vi "Base Card Passthrough(Relay).vi"(4 "Iterations":u32=50 min=1 max=64, 6 "Channels (1-64)":u16=64 min=1 max=64, 9 "Disconnection":enum16{"Open All", "Disconnect All"}(ring)=enum."Disconnect All", 11 "device":refnum<k21>="SET-2010-Mod2") -> (0 "error out":errorcluster, 1 "Disconnect Timing":T1, 2 "Connect Timing":T1)   [LabVIEW 2020, in "slsc-switch-benchmarks.lvlib"]
uses:
  slsc-switch-benchmarks.lvlib
  Timing Statistics.ctl
  <vilib>/SLSC_Switch/Relay Action.ctl
  <vilib>/SLSC_Switch/Initialize with Topology (Override Switches).vi
  <vilib>/SLSC_Switch/SLSC Switch.lvlib
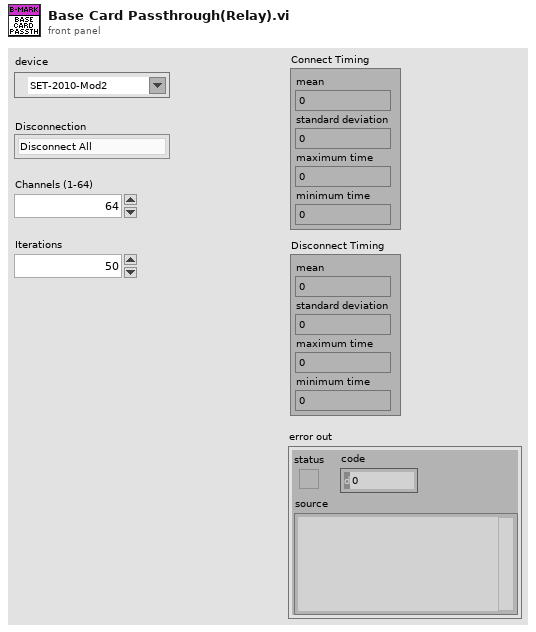
[diagram p1: front panel]
types:
  T1 = typedef "slsc-switch-benchmarks.lvlib/Timing Statistics.ctl" = cluster{"mean":dbl, "standard deviation":dbl, "maximum time":dbl, "minimum time":dbl}
  T2 = cluster{"Connect Time":dbl, "Disconnect Time":dbl}
  T3 = typedef "nislscslSession.ctl" = refnum<k20>
  T4 = cluster{"Connect Time":dbl, "Disconnect Time":dbl}[]
  T5 = typedef "SLSC Switch.lvlib/Relay Action.ctl" = i32
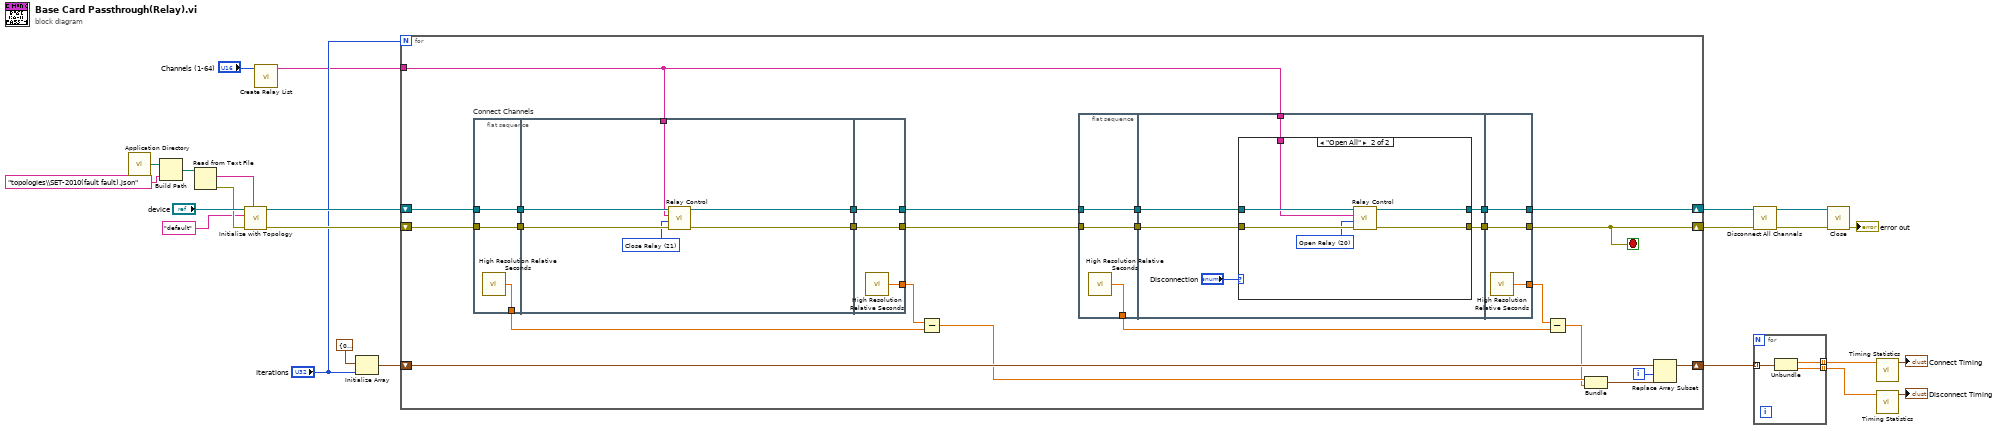
[diagram p0: block diagram]
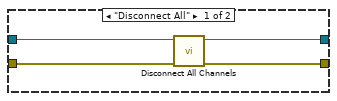
[diagram p2: hidden frame]
diagram:
  n1 = call <vilib>:"Application Directory.vi"() -> ("Application Directory"=w23:path)
  n2 = Build Path(base path=w23, name or relative path="topologies\\SET-2010(fault fault).json") -> (appended path=w21:path)
  n3 = Read from Text File(file (use dialog)=w21) -> (text=w19:string, error out=w20:errorcluster)  [unwired: 3 in, 2 out]
  n4 = call-poly <vilib>:"Initialize with Topology.vi"("switches json"=w19, "error in (no error)"=w20, "topology"="default", "device"="device") -> ("error out"=w16:errorcluster, "session out"=w17:T3)  [unwired: 6 in]
  n5 = call "Create Relay List.vi"("Channels (1-64)"="Channels (1-64)") -> ("Relay List"=w1:string)  [unwired: 10 in]
  n6 = Initialize Array(T2 {"Connect Time"=0.0, "Disconnect Time"=0.0}, "Iterations") -> (w12:T4)
  n7 = for {
    N: "Iterations" -> [_]
    shift-right: [w45] -> w11
    shift-left: w17 -> [w49]
    shift-right: [w32] -> w10
    shift-left: w16 -> [w48]
    shift-right: [w29] -> w7
    shift-left: w12 -> [w30]
    tunnel: w1 -> [w25]
    i -> [w31]
    stop <- w32 stop-if-true
    n8 = flat-sequence "Connect Channels" {
      tunnel: w48 -> [w73]
      tunnel: w49 -> [w74]
      tunnel: [w74] -> w42
      tunnel: [w73] -> w41
      tunnel: [w72] -> w39
      tunnel: [w78] -> w44
      tunnel: [w77] -> w43
      tunnel: w42 -> [w80]
      tunnel: w41 -> [w79]
      tunnel: w25 -> [w76]
      tunnel: [w82] -> w46
      tunnel: [w83] -> w47
      tunnel: w44 -> [w83]
      tunnel: w43 -> [w82]
      tunnel: [w81] -> w40
      frame #0 {
        n9 = call <vilib>:"High Resolution Relative Seconds.vi"() -> ("relative seconds"=w72:dbl)
      }
      frame #1 {
        w75 = T5 21 items=["Open Relay"=20, "Close Relay"=21] ("relay action (Close Relay)")
        n10 = call <vilib>:"Relay Control.vi"("error in (no error)"=w79, "relay action (Close Relay)"=w75, "relay names"=w76, "session in"=w80) -> ("error out"=w77:errorcluster, "session out"=w78:T3)  [unwired: 6 in]
      }
      frame #2 {
        n11 = call <vilib>:"High Resolution Relative Seconds.vi"() -> ("relative seconds"=w81:dbl)
      }
    }
    n12 = Subtract(x=w40, y=w39) -> (x-y=w28:dbl)
    n13 = flat-sequence {
      tunnel: w46 -> [w51]
      tunnel: w47 -> [w52]
      tunnel: [w52] -> w38
      tunnel: [w51] -> w37
      tunnel: [w50] -> w33
      tunnel: w38 -> [w58]
      tunnel: w37 -> [w57]
      tunnel: [w56] -> w36
      tunnel: [w55] -> w35
      tunnel: w25 -> [w53]
      tunnel: [w70] -> w45
      tunnel: [w71] -> w32
      tunnel: w36 -> [w71]
      tunnel: w35 -> [w70]
      tunnel: [w69] -> w34
      frame #0 {
        n14 = call <vilib>:"High Resolution Relative Seconds.vi"() -> ("relative seconds"=w50:dbl)
      }
      frame #1 {
        n15 = case shown="\"Open All\"" "Disconnection" {
          tunnel: w58 -> [w61 w68]
          tunnel: w57 -> [w62 w67]
          tunnel: [w59 w66] -> w56
          tunnel: [w60 w65] -> w55
          tunnel: w53 -> [_ w64]
          frame "Disconnect All" {
            n16 = call <vilib>:"Disconnect All Channels.vi"("error in (no error)"=w62, "session in"=w61) -> ("error out"=w59:errorcluster, "session out"=w60:T3)  [unwired: 8 in]
          }
          frame "Open All" {
            w63 = T5 20 items=["Open Relay"=20, "Close Relay"=21] ("relay action (Close Relay)")
            n17 = call <vilib>:"Relay Control.vi"("error in (no error)"=w67, "relay action (Close Relay)"=w63, "relay names"=w64, "session in"=w68) -> ("error out"=w66:errorcluster, "session out"=w65:T3)  [unwired: 6 in]
          }
        }
      }
      frame #2 {
        n18 = call <vilib>:"High Resolution Relative Seconds.vi"() -> ("relative seconds"=w69:dbl)
      }
    }
    n19 = Subtract(x=w34, y=w33) -> (x-y=w27:dbl)
    n20 = Bundle(w28, w27) -> (w26:cluster{dbl, dbl})  [unwired: 1 in]
    n21 = Replace Array Subset(array=w30, new element=w26, index=w31) -> (w29:T4)
  }
  n22 = call <vilib>:"Disconnect All Channels.vi"("error in (no error)"=w10, "session in"=w11) -> ("error out"=w9:errorcluster, "session out"=w8:T3)  [unwired: 8 in]
  n23 = for {
    tunnel: w7 -> [w86] mode=indexing
    tunnel: [w85] -> w6 mode=indexing
    tunnel: [w84] -> w5 mode=indexing
    n24 = Unbundle(w86) -> ("Connect Time"=w85:dbl, "Disconnect Time"=w84:dbl)
  }
  n25 = call <vilib>:"Close.vi"("error in (no error)"=w9, "session in"=w8) -> ("error out"=→"error out":errorcluster)  [unwired: 9 in]
  n26 = call "Timing Statistics.vi"("Execution Speeds"=w6) -> ("Timing Statistics"=→"Connect Timing":T1)  [unwired: 10 in]
  n27 = call "Timing Statistics.vi"("Execution Speeds"=w5) -> ("Timing Statistics"=→"Disconnect Timing":T1)  [unwired: 10 in]
